vi "scan_duration.vi"(1 "x-counter":i32, 2 "Time per Line":dbl) -> (0 "Duration (m.s)":string)   [LabVIEW 2020]
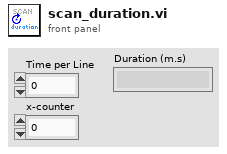
[diagram p1: front panel]
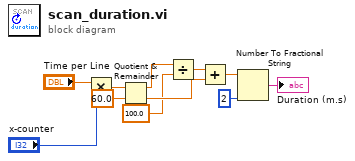
[diagram p0: block diagram]
diagram:
  n1 = Multiply(x="Time per Line", y="x-counter") -> (x*y=w5:dbl)
  n2 = Quotient & Remainder(x=w5, y=60.0) -> (x-y*floor(x/y)=w8:dbl, floor(x/y)=w10:dbl)
  n3 = Divide(x=w8, y=100.0) -> (x/y=w9:dbl)
  n4 = Add(x=w9, y=w10) -> (x+y=w6:dbl)
  n5 = Number To Fractional String(number=w6, precision (6)=i16 2) -> (F-format string=→"Duration (m.s)":string)  [unwired: 2 in]
